vi "Main.vi"() -> ()   [LabVIEW 2020]
uses:
  NI-6115 (PXIe-6368)/NI-6368 (PXIe).lvclass
  C:/Users/Thomas/Documents/YouTube Videos/Interfaces/Demo Code - Copy/Analogue Input/Analogue Input.lvclass
  NI-9381 (c series)/NI-9381 (c series).lvclass
  NI-9239 (C Series)/NI-9239 (C Series).lvclass
  Analogue Input/Analogue Input.lvclass
  PSU/AIO.lvclass
  Hardware/Instrument.lvclass
  DMM/Multifunction IO.lvclass
  C:/Users/Thomas/Documents/YouTube Videos/Interfaces/Demo Code - Copy/DMM/Multifunction IO.lvclass
panel:
  out "Events":string
  in  "Select":bool
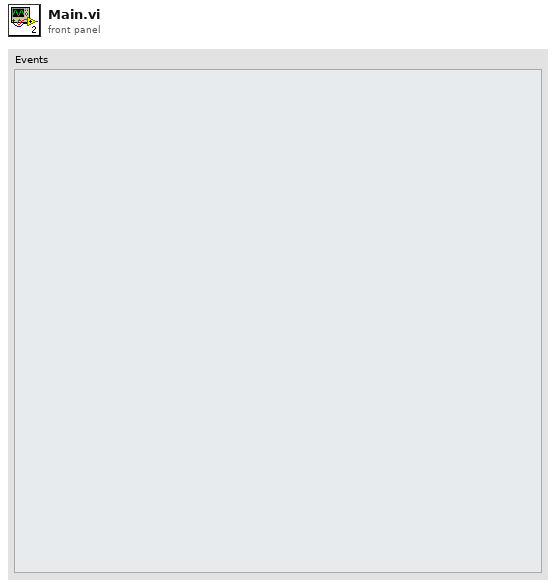
[diagram p1: front panel]
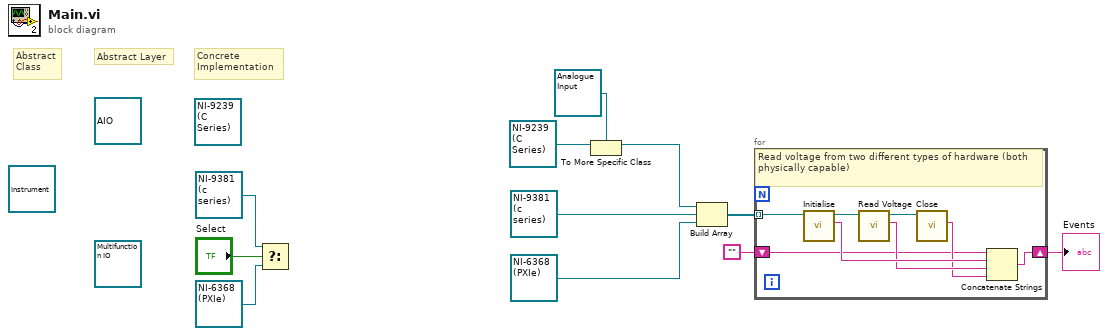
[diagram p0: block diagram]
diagram:
  (unwired) refnum<class "Multifunction IO.lvclass"> refnum ("Multifunction IO.lvclass")
  (unwired) refnum<class "Instrument.lvclass"> refnum ("Instrument.lvclass")
  (unwired) refnum<class "NI-9239 (C Series).lvclass"> refnum ("NI-9239.lvclass")
  (unwired) refnum<class "AIO.lvclass"> refnum ("AIO.lvclass")
  # "Concrete\nImplementation"
  # "Abstract\nClass"
  # "Abstract Layer"
  n1 = Select(t=refnum<class "NI-9381 (c series).lvclass"> refnum ("NI-9381 (c series).lvclass"), s="Select", f=refnum<class "NI-6368 (PXIe).lvclass"> refnum ("NI-6368 (PXIe).lvclass")) -> ()  [unwired: 1 out]
  n2 = To More Specific Class(target class=refnum<class "Analogue Input.lvclass"> refnum ("Analogue Input.lvclass"), reference=refnum<class "NI-9239 (C Series).lvclass"> refnum ("NI-9239.lvclass")) -> (specific class reference=w4:refnum<class "Analogue Input.lvclass">)  [unwired: 1 in, 1 out]
  n3 = Build Array(w4, refnum<class "NI-9381 (c series).lvclass"> refnum ("NI-9381 (c series).lvclass"), refnum<class "NI-6368 (PXIe).lvclass"> refnum ("NI-6368 (PXIe).lvclass")) -> (w8:refnum<class "Analogue Input.lvclass">[])
  n4 = for {
    tunnel: w8 -> [w19] mode=indexing
    shift-right: [w12] -> w1
    shift-left: "" -> [w13]
    # "Read voltage from two different types of hardware (both physically capable)"
    n5 = call-dynamic "Initialise.vi"("DAQ Types in"=w19) -> ("Status"=w16:string, "DAQ Types out"=w18:refnum<class "Analogue Input.lvclass">)  [unwired: 8 in, 1 out]
    n6 = call-dynamic "Read Voltage.vi"("Analogue Input in"=w18) -> ("Status"=w15:string, "Analogue Input out"=w17:refnum<class "Analogue Input.lvclass">)  [unwired: 8 in, 1 out]
    n7 = call-dynamic "Close.vi"("DAQ Types in"=w17) -> ("Status"=w14:string)  [unwired: 8 in, 2 out]
    n8 = Concatenate Strings(w13, w16, w15, w14) -> (w12:string)
  }
  "Events" <- w1
